vi "Keithley 6514 Data Format Config.vi"(0 "Resource In":refnum<visa-resource-name>, 1 "Check For SCPI Errors? (T)":bool=TRUE, 5 "Time (F)":bool, 7 "Status (F)":bool, 9 "Data Type (ASCII:0)":u16(ring) items=["ASCII", "Single Precision REAL"], 11 "error in (no error)":errorcluster, 12 "Binary Byte Order (Swapped:T))":bool=TRUE, 13 "Data Format for\nReading Status Registers (ASCII:0)":u16(ring) items=["ASCII", "Hexadecimal", "Octal", "Binary"], 14 "Data Format for\nReading Output Patterns (ASCII:0)":u16(ring) items=["ASCII", "Hexadecimal", "Octal", "Binary"]) -> (4 "Resource Out (dupl)":refnum<visa-resource-name>, 15 "error out":T1)   [LabVIEW 2010, in "Keithley 6514 LV 2009.lvlib"]
doc: "This VI is used to set the data format that will be used by the 6514 to return data over the GPIB bus. Certain elements are set to ON as the default.\n\nParameters:\nGPIB Address: Default to 14\n\nData Type:\n0 = ASCII\n1 = SREAL\n\nBinary Byte Order:\nFALSE = Normal\nTRUE = Swapped\n\nTime:\nFALSE = Off\nTRUE = On\n\nStatus:\nFALSE = Off\nTRUE = On\n\nData Format for Reading Status Registers:\n0 = ASCII\n1 = Hexadecimal\n2 = Octal\n3 = Binary\n\nData Format for Reading Output Patterns:\n0 = ASCII\n1 = Hexadecimal\n2 = Octal\n3 = Binary"
uses:
  Keithley 6514 LV 2009.lvlib
panel:
  # "SWAPPED\nNORMAL"
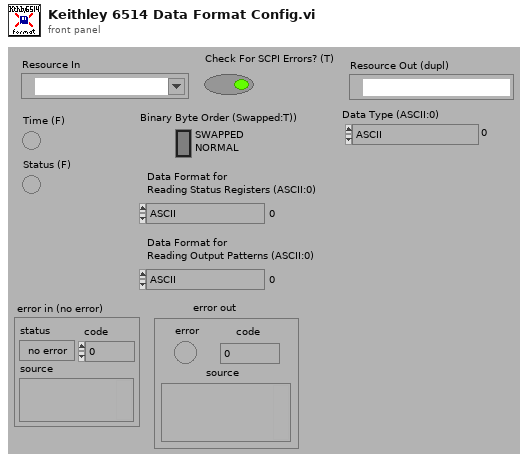
[diagram p1: front panel]
types:
  T1 = cluster{"error":bool, "code":i32, "source":string}
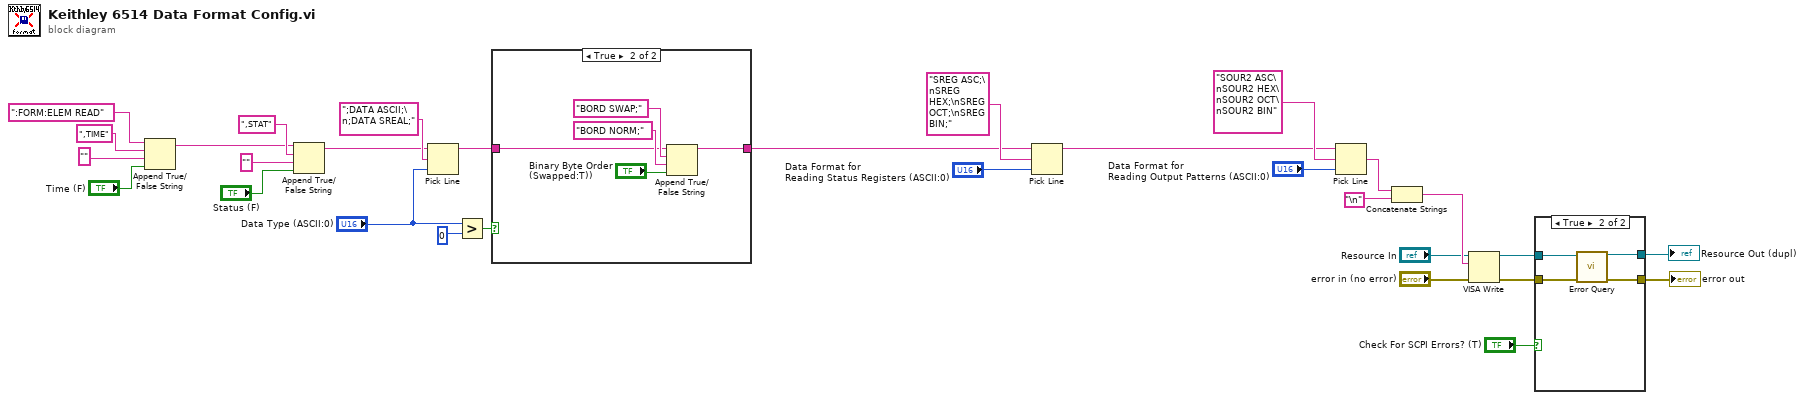
[diagram p0: block diagram]
diagram:
  n1 = Append True/False String(1:"Time (F)", 2:"", 3:",TIME", 4:":FORM:ELEM READ") -> (0:w19:string)
  n2 = Append True/False String(1:"Status (F)", 2:"", 3:",STAT", 4:w19) -> (0:w18:string)
  n3 = Pick Line(string ("")=w18, multi-line string=";DATA ASCII;\n;DATA SREAL;", line index="Data Type (ASCII:0)") -> (output string=w13:string)
  n4 = Greater?(x="Data Type (ASCII:0)", y=u16 0) -> (0:w27:bool)
  n5 = case shown="True" w27 {
    tunnel: w13 -> [w31 w33]
    tunnel: [w31 w32] -> w12
    frame False {
    }
    frame True {
      n6 = Append True/False String(1:"Binary Byte Order (Swapped:T))", 2:"BORD NORM;", 3:"BORD SWAP;", 4:w33) -> (0:w32:string)
    }
  }
  n7 = Pick Line(string ("")=w12, multi-line string="SREG ASC;\nSREG HEX;\nSREG OCT;\nSREG BIN;", line index="Data Format for\nReading Status Registers (ASCII:0)") -> (output string=w11:string)
  n8 = Pick Line(string ("")=w11, multi-line string="SOUR2 ASC\nSOUR2 HEX\nSOUR2 OCT\nSOUR2 BIN", line index="Data Format for\nReading Output Patterns (ASCII:0)") -> (output string=w10:string)
  n9 = Concatenate Strings(w10, "\n") -> (w8:string)
  n10 = VISA Write(VISA resource name="Resource In", write buffer=w8, error in (no error)="error in (no error)") -> (VISA resource name out=w4:refnum<visa-resource-name>, error out=w3:errorcluster)  [unwired: 1 out]
  n11 = case shown="True" "Check For SCPI Errors? (T)" {
    tunnel: w4 -> [w38 w42]
    tunnel: w3 -> [w37 w41]
    tunnel: [w38 w40] -> w2
    tunnel: [w37 w39] -> w1
    frame False {
    }
    frame True {
      n12 = call "Error Query.vi"("VISA Resource In"=w42, "error in (no error)"=w41) -> ("VISA Resource Out (dupl)"=w40:refnum<visa-resource-name>, "error out"=w39:errorcluster)  [unwired: 10 in, 2 out]
    }
  }
  "error out" <- w1
  "Resource Out (dupl)" <- w2
